vi "Get_Power_Unit.vi"(8 "error in (no error)":errorcluster, 11 ".NET Reference in":refnum<k24>) -> (0 "error out":errorcluster, 2 "unit":enum16{"dBm", "mW", ""}(ring), 3 "Reference out":refnum<k24>)   [LabVIEW 2017]
uses:
  D:/test/FULLband-sts/Fullband_Sample/DLL/InstrumentDLL.dll
  DLL/InstrumentDLL.dll
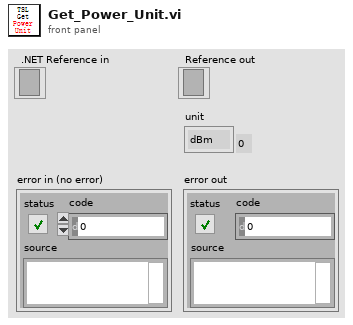
[diagram p1: front panel]
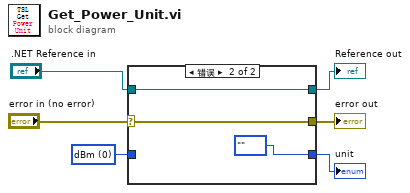
[diagram p0: block diagram]
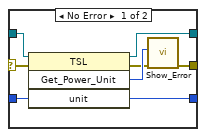
[diagram p2: hidden frame]
diagram:
  w3 = 0 items=["dBm", "mW"] ("unit")
  n1 = case shown="错误" "error in (no error)" {
    selector: "error in (no error)" -> [w7 w17]
    tunnel: ".NET Reference in" -> [w14 w16]
    tunnel: [w13 w16] -> w5
    tunnel: [w8 w17] -> w4
    tunnel: w3 -> [w12 _]
    tunnel: [w11 enum16{"dBm", "mW", ""}."" ("unit")] -> w2
    frame No Error {
      n2 = invoke on="调用节点" class="TSL" method="Get_Power_Unit"(reference=w14, error in=w7, "unit"=w12) -> (reference out=w13:refnum<k24>, error out=w9:errorcluster, "Get_Power_Unit"=w10:i32, "unit"=w11:i32)  [unwired: 1 in]
      n3 = call "Show_Error.vi"("error in (no error)"=w9, "Error"=w10) -> ("error out"=w8:errorcluster)  [unwired: 9 in]
    }
    frame Error {
    }
  }
  "Reference out" <- w5
  "error out" <- w4
  "unit" <- w2
